vi "TEST_NT_HELPER_DBL.vi"() -> ()   [LabVIEW 2023]
uses:
  <vilib>/Rock Robotics/Network Tables/NT Read Number.vi
  <vilib>/Rock Robotics/Network Tables/NT Write Number.vi
panel:
  out "value 2":dbl
  out "value":dbl
  in  "name 2":string="Test4150Val1"
  in  "name":string="Test4150Val2"
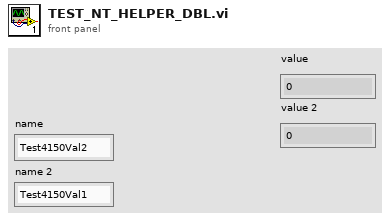
[diagram p1: front panel]
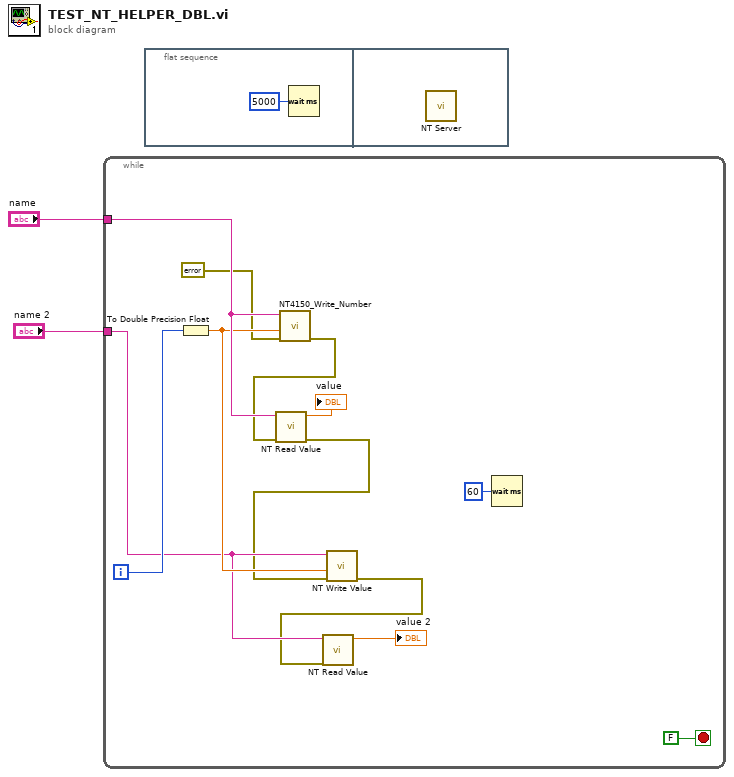
[diagram p0: block diagram]
diagram:
  n1 = while {
    tunnel: "name" -> [w14]
    tunnel: "name 2" -> [w10]
    i -> [w12]
    stop <- FALSE stop-if-true
    n2 = To Double Precision Float(number=w12) -> (double precision float=w11:dbl)
    n3 = call "NT4150_Write_Number.vi"("error in"=errorcluster {"status"=FALSE, "code"=0, "source"=""}, "value"=w11, "name"=w14) -> ("error out"=w9:errorcluster)  [unwired: 8 in]
    n4 = call-poly <vilib>:"NT Read Value.vi"("error in"=w9, "name"=w14) -> ("error out"=w8:errorcluster, "value"=→"value":dbl)  [unwired: 7 in, 1 out]
    n5 = call-poly <vilib>:"NT Write Value.vi"("error in"=w8, "value"=w11, "name"=w10) -> ("error out"=w7:errorcluster)  [unwired: 8 in]
    n6 = call-poly <vilib>:"NT Read Value.vi"("error in"=w7, "name"=w10) -> ("value"=→"value 2":dbl)  [unwired: 7 in, 2 out]
    n7 = Wait (ms)(milliseconds to wait=u32 60) -> ()  [unwired: 1 out]
  }
  n8 = flat-sequence {
    frame #0 {
      n9 = Wait (ms)(milliseconds to wait=u32 5000) -> ()  [unwired: 1 out]
    }
    frame #1 {
      n10 = call <vilib>:"NT Server.vi"() -> ()  [unwired: 11 in, 1 out]
    }
  }
